vi "FS Functions.vi"   [LabVIEW 2019]
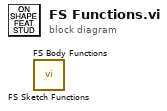
[diagram p0: block diagram]
diagram:
  n1 = call "FS Sketch Functions.vi"() -> ()  [unwired: 11 in, 1 out]
  n2 = call "FS Body Functions.vi"() -> ()  [unwired: 11 in, 1 out]
